vi "Drive Commands.vi"() -> ()   [LabVIEW 2012]
panel:
  in  "Drive Commands":T1
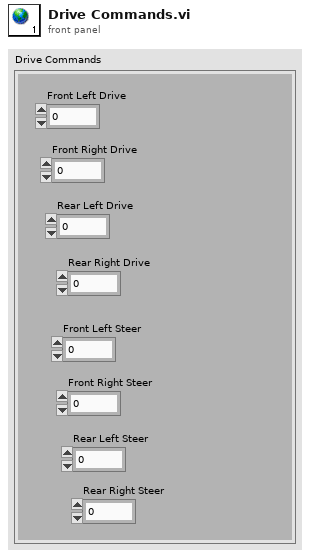
[diagram p1: front panel]
types:
  T1 = cluster{"Front Left Drive":dbl, "Front Right Drive":dbl, "Rear Left Drive":dbl, "Rear Right Drive":dbl, "Front Left Steer":dbl, "Front Right Steer":dbl, "Rear Left Steer":dbl, "Rear Right Steer":dbl}
diagram:
